vi "SauvTempTlog.vi"(6 "Chauffage":dbl, 7 "CheminSauv":path=path "C:/Données/Run003" caption="Fichier de Sauvegarde", 8 "error in":errorcluster, 9 "NiveauHe":dbl, 10 "DonnéesY":dbl[](array[numeric]), 11 "NouvTemps":dbl) -> (0 "error out":errorcluster, 1 "NiveauHe Out":dbl, 2 "DonnéesY out":dbl[](array[numeric]), 3 "NouvTemps Out":dbl, 4 "Chauffage Out":dbl)   [LabVIEW 2010]
doc: "Ce Vi sauvegarde les données sous forme de collonnes dans le fichier texte de sauvegarde"
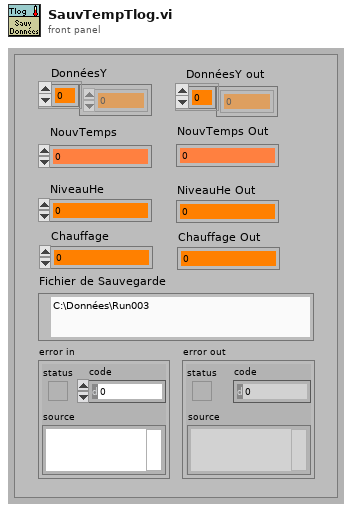
[diagram p1: front panel]
types:
  T1 = enum16{"open", "open or create", "create or replace", "create", "open (read only)"}
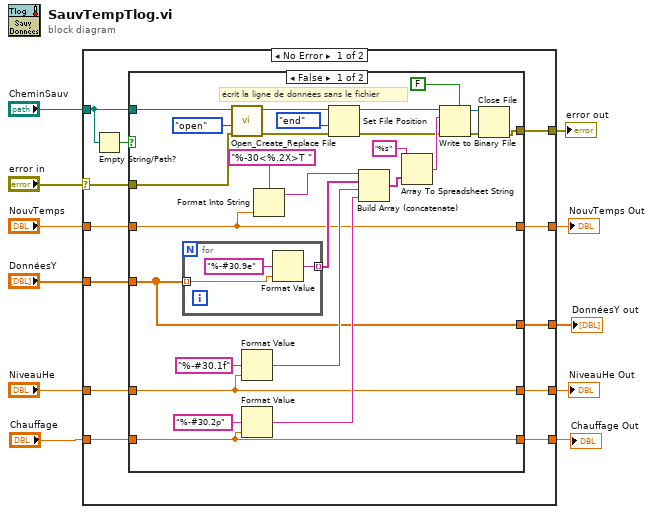
[diagram p0: block diagram]
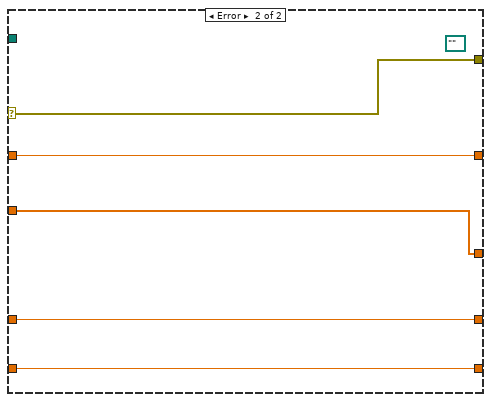
[diagram p3: hidden frame]
diagram:
  n1 = case shown="No Error" "error in" {
    selector: "error in" -> [w22 w62]
    tunnel: [w23 w62] -> w11
    tunnel: "CheminSauv" -> [w16 _]
    tunnel: "DonnéesY" -> [w20 w60]
    tunnel: "NouvTemps" -> [w21 w59]
    tunnel: "NiveauHe" -> [w19 w61]
    tunnel: [w12 w59] -> w5
    tunnel: [w13 w60] -> w4
    tunnel: [w14 w61] -> w3
    tunnel: "Chauffage" -> [w18 w58]
    tunnel: [w15 w58] -> w1
    frame No Error {
      n2 = Empty String/Path?(string/path=w16) -> (empty?=w17:bool)
      n3 = case shown="False" w17 {
        tunnel: [w44 w57] -> w23
        tunnel: w22 -> [w43 w57]
        tunnel: w16 -> [w42 _]
        tunnel: w21 -> [w24 w56]
        tunnel: w20 -> [w30 w55]
        tunnel: w19 -> [w31 w54]
        tunnel: w18 -> [w32 w53]
        tunnel: [w32 w53] -> w15
        tunnel: [w31 w54] -> w14
        tunnel: [w30 w55] -> w13
        tunnel: [w24 w56] -> w12
        frame False {
          # "écrit la ligne de données sans le fichier"
          n4 = for {
            tunnel: w30 -> [w51] mode=indexing
            tunnel: [w50] -> w39 mode=indexing
            n5 = Format Value(format string="%-#30.9e", value (0)=w51) -> (output string=w50:string)  [unwired: 1 in]
          }
          n6 = call <vilib>:"Open_Create_Replace File.vi"("error in (no error)"=w43, "function (open:0)"=T1."open", "file path"=w42) -> ("error out"=w49:errorcluster, "refnum"=w45:refnum<file>)  [unwired: 5 in, 2 out]
          n7 = Format Value(format string="%-#30.1f", value (0)=w31) -> (output string=w38:string)  [unwired: 1 in]
          n8 = Format Value(format string="%-#30.2p", value (0)=w32) -> (output string=w33:string)  [unwired: 1 in]
          n9 = Format Into String(format string="%-30<%.2X>T " ("chaîne de format"), w24) -> (resulting string=w25:string)  [unwired: 2 in, 1 out]
          n10 = Set File Position(refnum=w45, from (0:start)=enum16{"start", "end", "current"}."end" ("pos mode (0:2)"), error in=w49) -> (refnum out=w29:refnum<file>, error out=w28:errorcluster)  [unwired: 1 in]
          n11 = Build Array (concatenate)(w25, w39, w38, w33) -> (w37:string[])
          n12 = Array To Spreadsheet String(array=w37, 3:"%s" ("format string")) -> (spreadsheet string=w35:string)  [unwired: 1 in]
          n13 = Write to Binary File(file (use dialog)=w29, data=w35, error in=w28, 5:FALSE ("ajouter une taille de tableau ou de chaîne ? (V)")) -> (refnum out=w46:refnum<file>, error out=w48:errorcluster)  [unwired: 2 in, 1 out]
          n14 = Close File(refnum=w46, error in=w48) -> (error out=w44:errorcluster)  [unwired: 1 out]
        }
        frame True {
          # "path vide: on ne sauvegarde pas"
        }
      }
    }
    frame Error {
      (unwired) path "" ("path")
    }
  }
  "error out" <- w11
  "NouvTemps Out" <- w5
  "DonnéesY out" <- w4
  "NiveauHe Out" <- w3
  "Chauffage Out" <- w1
